vi "SetIOPinPol.vi"(8 "错误输入（无错误）":errorcluster, 9 "SelPinType":i32, 10 "闸门跟踪属性":u8, 11 "SelPinNum":i32) -> (0 "错误输出":errorcluster)   [LabVIEW 2014]
uses:
  X86Dll/ZXUTConfigMgr.dll
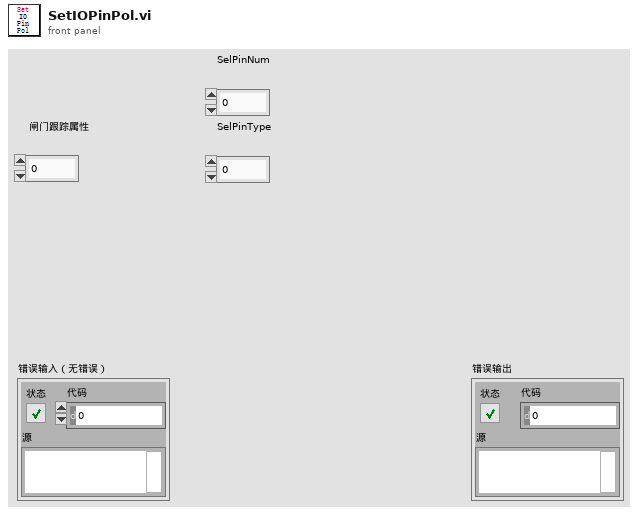
[diagram p1: front panel]
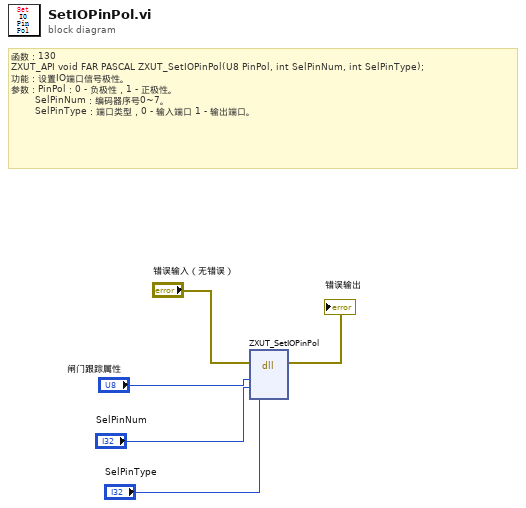
[diagram p0: block diagram]
diagram:
  # "函数：130\nZXUT_API void\tFAR PASCAL ZXUT_SetIOPinPol(U8 PinPol, int SelPinNum, int SelPinType);\n功能：设置IO端口信号极性。\n参数：PinPol：0 - 负极性，1 - 正极性。\n        SelPinNum：编码器序号0~7。\n        SelPinType：端口类型，0 - 输入端口 1 - 输出端口。"
  n1 = dll-call lib="D:/Software/Utrasonic on-line monitoring/X86Dll/ZXUTConfigMgr.dll" fn="ZXUT_SetIOPinPol"(error in="错误输入（无错误）", "PinPol"="闸门跟踪属性", "SelPinNum"="SelPinNum", "SelPinType"="SelPinType") -> (error out=→"错误输出":errorcluster)  [unwired: 6 in, 1 out]
